vi "multiColorWormMoleculeSettings.vi"(0 "molecule":string) -> (1 "laserWavelength":dbl, 2 "filter wheel position":u8, 3 "laser power (mW)":dbl, 4 "exposure time (s)":dbl, 5 "exposureTimeMultiplier":dbl, 6 "slider position":u16)   [LabVIEW 2017]
uses:
  globalUtilities.vi
panel:
  # "Returns indexes of filter wheel and slider/shutter position\ngiven the molecule."
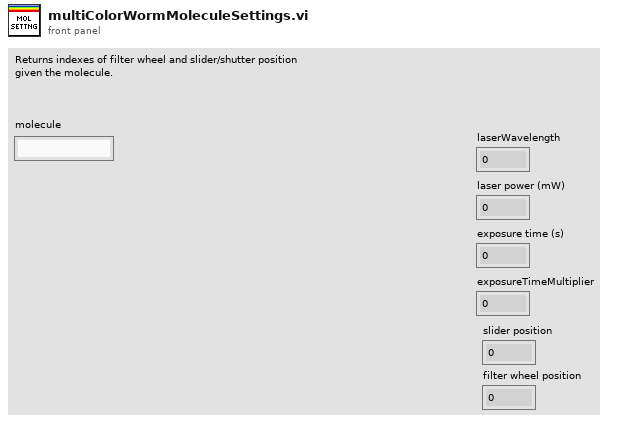
[diagram p1: front panel]
types:
  T1 = cluster{"laserWavelength":dbl, "exposureTime":dbl, "filterWheelPosition":u8, "name":string, "exposureTimeMultiplier":dbl}[]
  T2 = cluster{"laserWavelength (nm)":dbl, "laserPower (mW)":dbl, "sliderPosition":u16}[]
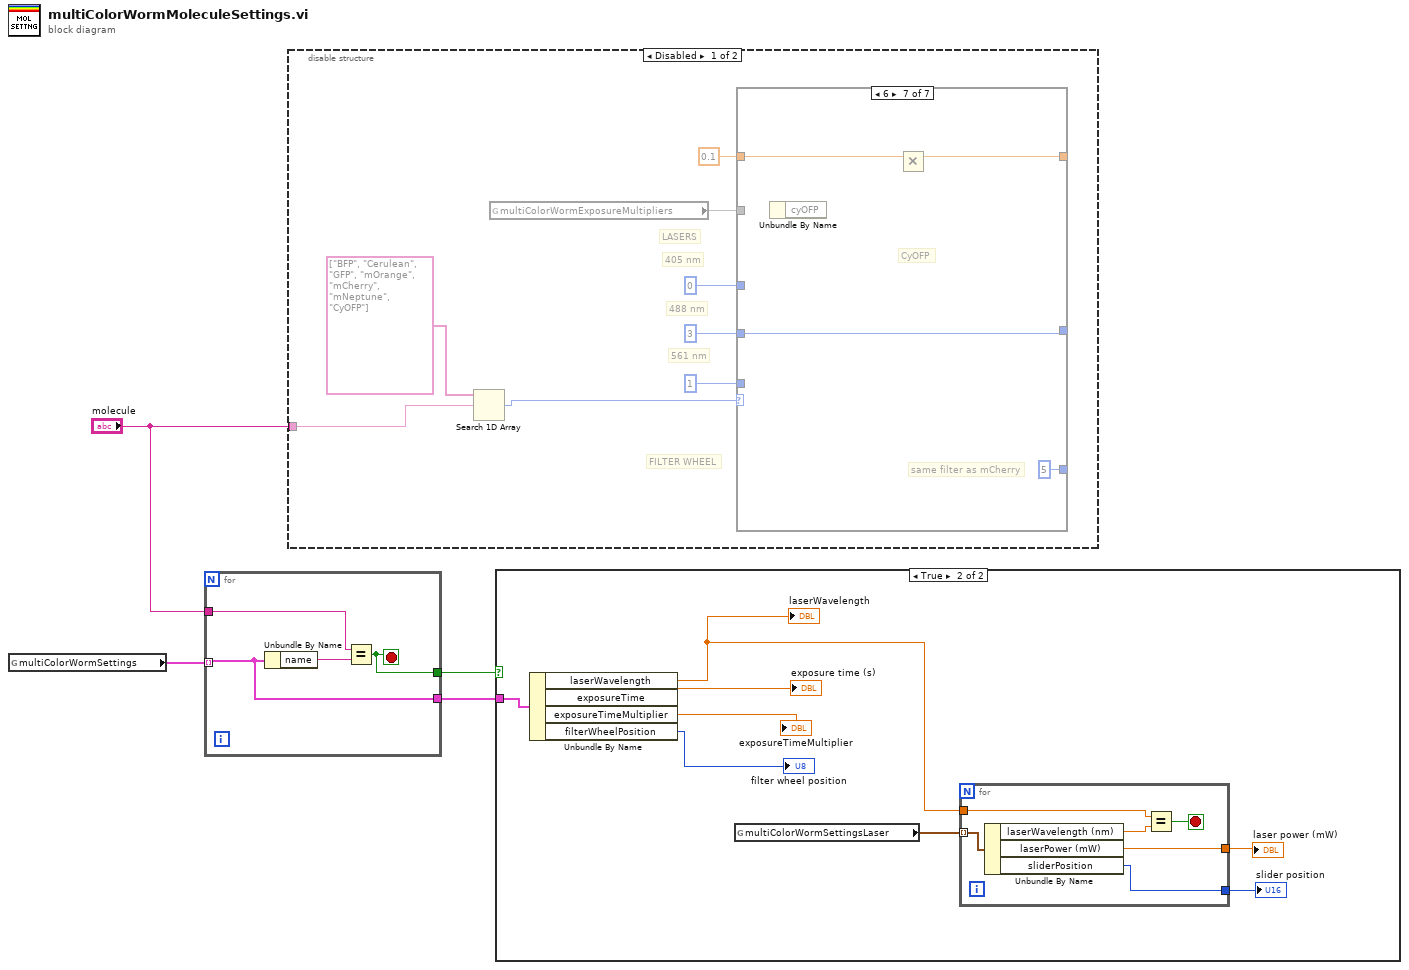
[diagram p0: block diagram]
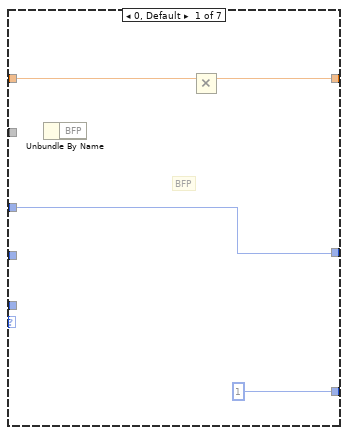
[diagram p2: hidden frame]
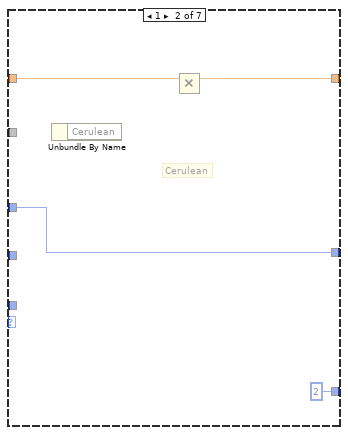
[diagram p3: hidden frame]
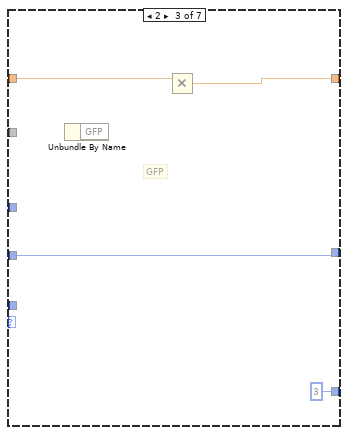
[diagram p4: hidden frame]
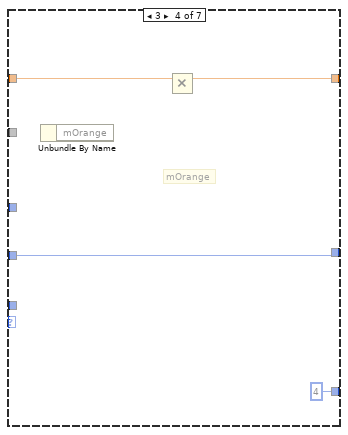
[diagram p5: hidden frame]
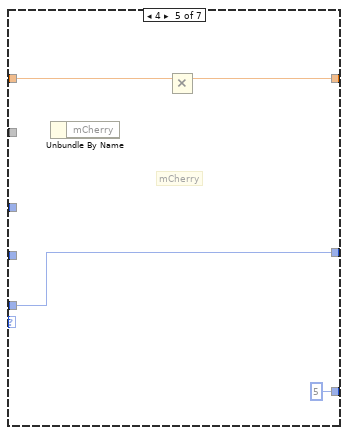
[diagram p6: hidden frame]
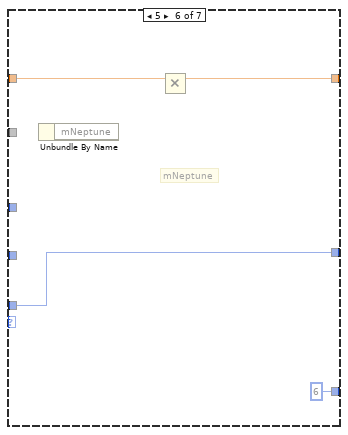
[diagram p7: hidden frame]
diagram:
  n1 = global read "globalUtilities.vi" "multiColorWormSettings"() -> (w3:T1)
  n2 = for {
    tunnel: "molecule" -> [w7]
    tunnel: w3 -> [w6] mode=indexing
    tunnel: [w6] -> w1
    tunnel: [w5] -> w2
    stop <- w5 stop-if-true
    n3 = Unbundle By Name(w6) -> ("name"=w8:string)
    n4 = Equal?(x=w7, y=w8) -> (x = y?=w5:bool)
  }
  n5 = disable-structure shown="Disabled" {
    disable-tunnel: "molecule" -> [w9 _]
    frame Disabled {
      # "FILTER WHEEL"
      # "LASERS"
      # "561 nm"
      # "488 nm"
      # "405 nm"
      n6 = Search 1D Array(1D array=string[] ["BFP", "Cerulean", "GFP", "mOrange", "mCherry", "mNeptune", "CyOFP"], element=w9) -> (index of element=w10:i32)  [unwired: 1 in]
      n7 = global read "globalUtilities.vi" "multiColorWormExposureMultipliers"() -> (w11)
      n8 = case shown="6" w10 {
        tunnel: 0 -> [w20 w24 _ _ _ _ _]
        tunnel: 3 -> [_ _ w28 w32 _ _ w43]
        tunnel: 1 -> [_ _ _ _ w35 w39 _]
        tunnel: [w20 w24 w28 w32 w35 w39 w43] -> _
        tunnel: [1 2 3 4 5 6 5] -> _
        tunnel: 0.1 -> [w18 w22 w25 w30 w34 w38 w42]
        tunnel: [w17 w21 w26 w29 w33 w37 w41] -> _
        tunnel: w11 -> [_ _ _ _ _ _ _]
        frame 0, Default {
          # "BFP"
          n9 = Unbundle By Name() -> ()  [unwired: 1 in, 1 out]
          n10 = Multiply(x=w18) -> (x*y=w17:dbl)  [unwired: 1 in]
        }
        frame 1 {
          # "Cerulean"
          n11 = Unbundle By Name() -> ()  [unwired: 1 in, 1 out]
          n12 = Multiply(x=w22) -> (x*y=w21:dbl)  [unwired: 1 in]
        }
        frame 2 {
          # "GFP"
          n13 = Unbundle By Name() -> ()  [unwired: 1 in, 1 out]
          n14 = Multiply(x=w25) -> (x*y=w26:dbl)  [unwired: 1 in]
        }
        frame 3 {
          # "mOrange"
          n15 = Unbundle By Name() -> ()  [unwired: 1 in, 1 out]
          n16 = Multiply(x=w30) -> (x*y=w29:dbl)  [unwired: 1 in]
        }
        frame 4 {
          # "mCherry"
          n17 = Unbundle By Name() -> ()  [unwired: 1 in, 1 out]
          n18 = Multiply(x=w34) -> (x*y=w33:dbl)  [unwired: 1 in]
        }
        frame 5 {
          # "mNeptune"
          n19 = Unbundle By Name() -> ()  [unwired: 1 in, 1 out]
          n20 = Multiply(x=w38) -> (x*y=w37:dbl)  [unwired: 1 in]
        }
        frame 6 {
          # "same filter as mCherry"
          # "CyOFP"
          n21 = Unbundle By Name() -> ()  [unwired: 1 in, 1 out]
          n22 = Multiply(x=w42) -> (x*y=w41:dbl)  [unwired: 1 in]
        }
      }
    }
    frame Enabled {
    }
  }
  n23 = case shown="True" w2 {
    tunnel: w1 -> [_ w52]
    frame False {
    }
    frame True {
      n24 = Unbundle By Name(w52) -> ("laserWavelength"=w48:dbl, "exposureTime"=→"exposure time (s)":dbl, "exposureTimeMultiplier"=→"exposureTimeMultiplier":dbl, "filterWheelPosition"=→"filter wheel position":u8)
      "laserWavelength" <- w48
      n25 = global read "globalUtilities.vi" "multiColorWormSettingsLaser"() -> (w49:T2)
      n26 = for {
        tunnel: w49 -> [w58] mode=indexing
        tunnel: w48 -> [w56]
        tunnel: [w54] -> w47
        tunnel: [w53] -> w46
        stop <- w55 stop-if-true
        n27 = Unbundle By Name(w58) -> ("laserWavelength (nm)"=w57:dbl, "laserPower (mW)"=w54:dbl, "sliderPosition"=w53:u16)
        n28 = Equal?(x=w56, y=w57) -> (x = y?=w55:bool)
      }
      "slider position" <- w46
      "laser power (mW)" <- w47
    }
  }
